vi "Find Alias.vi"(10 "VI Ref":refnum<vi>) -> (2 "Alias":string)   [LabVIEW 2020, in "jettl.lvlib" / "Actor.lvlib"]
uses:
  Actor.lvlib
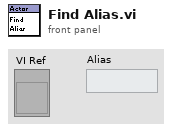
[diagram p1: front panel]
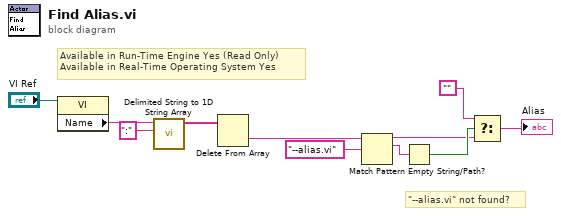
[diagram p0: block diagram]
diagram:
  # "Available in Run-Time Engine Yes (Read Only) \nAvailable in Real-Time Operating System Yes"
  # "\"--alias.vi\" not found?"
  n1 = property class="VI"(reference="VI Ref") -> ("Name"=w6:string)  [unwired: 1 in, 2 out]
  n2 = call <vilib>:"Delimited String to 1D String Array.vi"("delimiter"=":", "delimited string"=w6) -> ("string array"=w8:string[])  [unwired: 9 in]
  n3 = Delete From Array "Delete From Array"(array=w8) -> (deleted portion=w7:string)  [unwired: 2 in, 1 out]
  n4 = Match Pattern(string=w7, regular expression="--alias.vi") -> (before substring=w3:string, match substring=w10:string)  [unwired: 1 in, 2 out]
  n5 = Empty String/Path?(string/path=w10) -> (empty?=w4:bool)
  n6 = Select(t="", s=w4, f=w3) -> (s? t:f=→"Alias":string)
